vi "Configure Sys (To) Clock Out.vi"(8 "error in (no error)":errorcluster, 10 "Clock Out (0: To Pulse)":T1(ring), 11 "VISA resource name":refnum<visa-resource-name>) -> (0 "error out":errorcluster, 3 "VISA resource name out":refnum<visa-resource-name>)   [LabVIEW 2012, in "Quantum Composers 9000 Series.lvlib"]
doc: "This VI is used to configure the external clock output. A value of \"To Pulse\" produces a pulse at each To period. Otherwise, a 50% duty cycle clock is generated with the indicated frequency."
uses:
  <instrlib>/Quantum Composers 9000 Series/Quantum Composers 9000 Series.lvlib
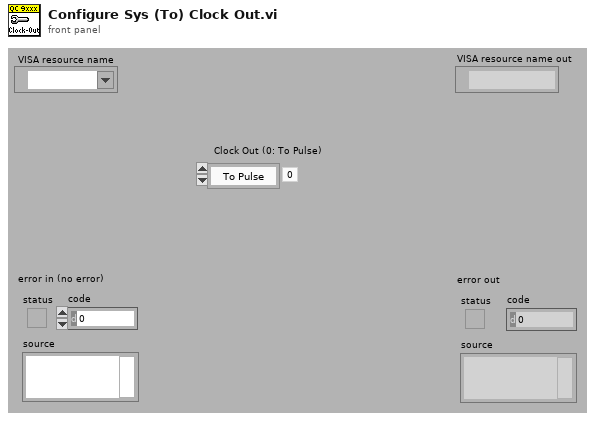
[diagram p1: front panel]
types:
  T1 = enum16{"To Pulse", "10 MHz", "11 MHz", "12 MHz", "14 MHz", "16 MHz", "20 MHz", "25 MHz", "33 MHz", "50 MHz", "100 MHz"}
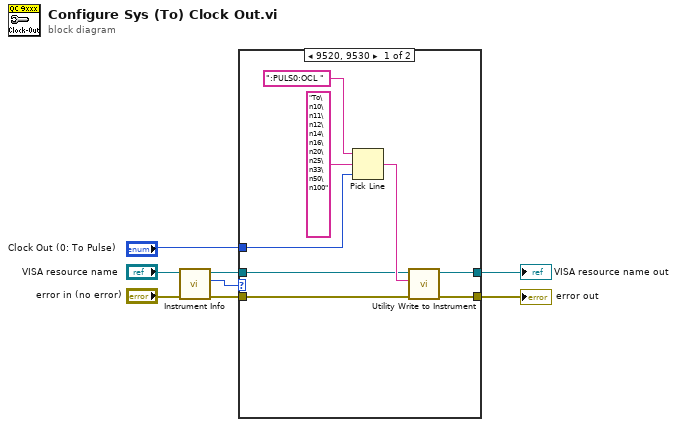
[diagram p0: block diagram]
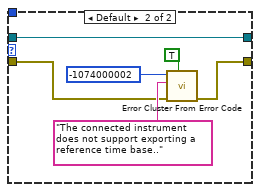
[diagram p2: hidden frame]
diagram:
  n1 = call <instrlib>:"Instrument Info.vi"("error in (no error)"="error in (no error)", "VISA resource name"="VISA resource name") -> ("error out"=w3:errorcluster, "Instr Model"=w4:u32, "VISA resource name out"=w5:refnum<visa-resource-name>)  [unwired: 6 in, 1 out]
  n2 = case shown="9520, 9530" w4 {
    tunnel: [w13 w22] -> w8
    tunnel: [w12 w17] -> w7
    tunnel: "Clock Out (0: To Pulse)" -> [w11 _]
    tunnel: w3 -> [w10 w18]
    tunnel: w5 -> [w9 w22]
    frame 9520, 9530 {
      n3 = Pick Line(string ("")=":PULS0:OCL ", multi-line string="To\n10\n11\n12\n14\n16\n20\n25\n33\n50\n100", line index=w11) -> (output string=w16:string)
      n4 = call <instrlib>:"Utility Write to Instrument.vi"("error in (no error)"=w10, "Write Buffer"=w16, "VISA resource name"=w9) -> ("error out"=w12:errorcluster, "VISA resource name out"=w13:refnum<visa-resource-name>)  [unwired: 6 in, 1 out]
    }
    frame Default {
      n5 = call <vilib>:"Error Cluster From Error Code.vi"("show call chain? (False)"=TRUE, "error in (no error)"=w18, "error message (\"\")"="The connected instrument does not support exporting a reference time base.." ("Source (VI Name)"), "error code (0)"=-1074000002 ("Code")) -> ("error out"=w17:errorcluster)  [unwired: 5 in]
    }
  }
  "error out" <- w7
  "VISA resource name out" <- w8
